vi "Open.vi"(8 "error in (no error)":errorcluster caption="entrée d'erreur (pas d'erreur)", 11 "Class LED Analyser in":refnum<class "Class LED Analyser FEASA.lvclass">) -> (0 "error out":errorcluster caption="sortie d'erreur", 3 "Class LED Analyser Out":refnum<class "Class LED Analyser FEASA.lvclass">)   [LabVIEW 2020, in "Library Instrument & Equipement.lvlib" / "Library LED Analyser.lvlib" / "Class LED Analyser FEASA.lvclass"]
uses:
  Class LED Analyser FEASA.lvclass
  C:/Users/ngarcin/OneDrive - Altyor/Standard TB/Class/LED Analyser/Class Led Analyser (Default)/Class LED Analyser (Default).lvclass
  Class LED Analyser FEASA.lvclass/Class LED Analyser FEASA.ctl
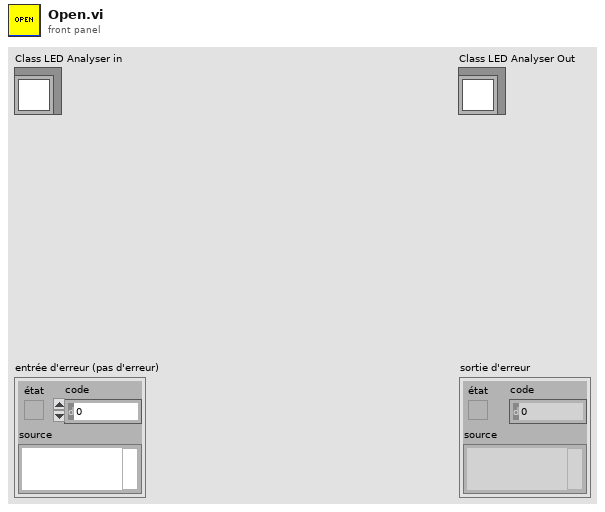
[diagram p1: front panel]
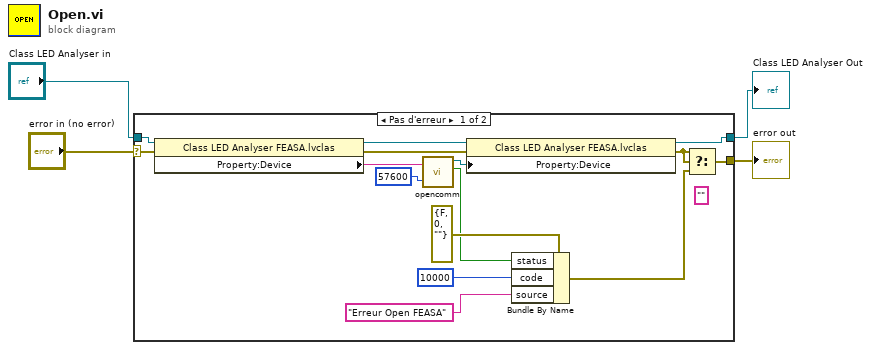
[diagram p0: block diagram]
diagram:
  n1 = case shown="Pas d'erreur" "error in (no error)" {
    selector: "error in (no error)" -> [w6 w21]
    tunnel: [w18 w21] -> w3
    tunnel: [w7 w20] -> w1
    tunnel: "Class LED Analyser in" -> [w19 w20]
    frame No Error {
      (unwired) "" ("Device")
      n2 = property class="Class LED Analyser FEASA.lvclas"(reference=w19, error in=w6) -> (reference out=w9:refnum<class "Class LED Analyser FEASA.lvclass">, error out=w10:errorcluster, "Property:Device"=w11:string)
      n3 = call "opencomm.vi"("VISA resource name"=w11, "Baud-rate (57600)"=u32 57600) -> ("duplicate VISA resource name"=w8:refnum<visa-resource-name>, "Error"=w16:bool)  [unwired: 2 in]
      n4 = property class="Class LED Analyser FEASA.lvclas"(reference=w9, error in=w10, "Property:Device"=w8) -> (reference out=w7:refnum<class "Class LED Analyser FEASA.lvclass">, error out=w5:errorcluster)
      n5 = Bundle By Name(cluster=errorcluster {"status"=FALSE, "code"=0, "source"=""} ("error IO"), "status"=w16, "code"=10000, "source"="Erreur Open FEASA") -> (w13:errorcluster)
      n6 = Select(t=w5, s=w5, f=w13) -> (s? t:f=w18:errorcluster)
    }
    frame Error {
    }
  }
  "error out" <- w3
  "Class LED Analyser Out" <- w1
